vi "RP Lockin Fast Continuous Sweeper.vi"(6 "Samples per read":i32=1024, 7 "Desimate result":i32, 8 "Error In":errorcluster, 9 "milliseconds to wait":u32=10, 10 "Frequencies":dbl[](array[numeric]), 11 "connection ID":refnum<k5>) -> (0 "Error Out":errorcluster, 1 "Y":dbl[](array[numeric]), 2 "X":dbl[](array[numeric]), 3 "connection ID out":refnum<k5>, 4 "F":dbl[](array[numeric]))   [LabVIEW 2015]
panel:
  out "Input Fifo cnt 2":i32
  out "32bit integer":i32
  out "Output Fifo cnt":i32
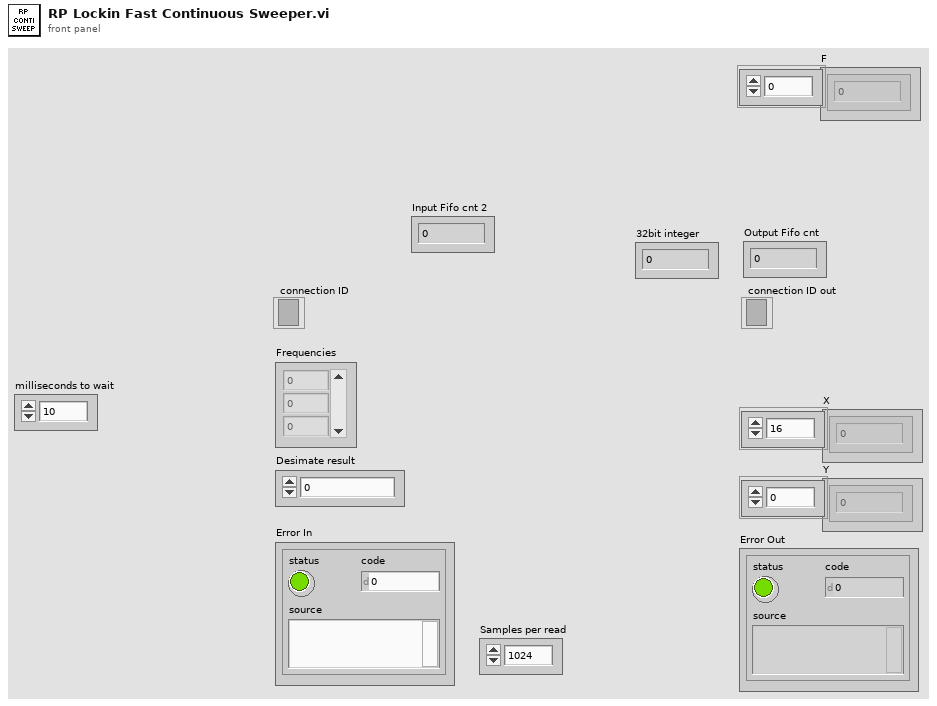
[diagram p1: front panel]
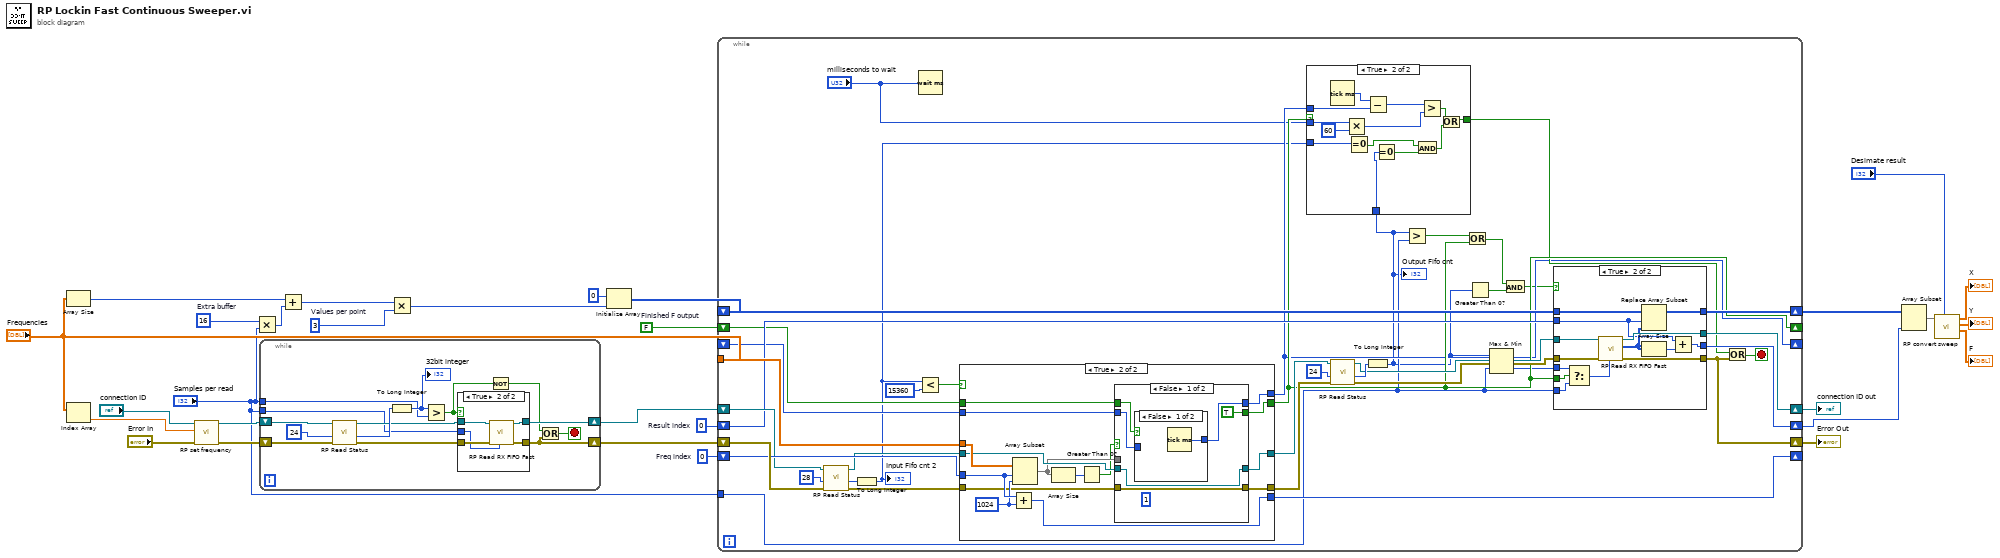
[diagram p0: block diagram]
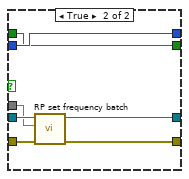
[diagram p6: hidden frame]
diagram:
  w13 = 3  # Values per point
  w16 = 16  # Extra buffer
  w19 = FALSE  # Finished F output
  w21 = 0  # Freq index
  w9 = 0  # Result index
  n1 = Array Size(array="Frequencies") -> (size(s)=w17:i32)
  n2 = Index Array(array="Frequencies") -> (element=w29:dbl)  [unwired: 1 in]
  n3 = call "RP set frequency.vi"("Error In"="Error In", "Frequency"=w29, "connection ID"="connection ID") -> ("Error Out"=w23:errorcluster, "connection ID out"=w25:refnum<k5>)  [unwired: 6 in, 1 out]
  n4 = Multiply(x=w16, y="Samples per read") -> (x*y=w15:i32)
  n5 = while {
    tunnel: "Samples per read" -> [w40]
    shift-right: [w30] -> w22
    shift-left: w23 -> [w37]
    shift-right: [w35] -> w24
    shift-left: w25 -> [w36]
    tunnel: "Samples per read" -> [w34]
    stop <- w33 stop-if-true
    n6 = call "RP Read Status.vi"("Error In"=w37, "Status offset"=u64 24, "connection ID"=w36) -> ("Error Out"=w32:errorcluster, "Status response"=w41:u32, "connection ID out"=w39:refnum<k5>)  [unwired: 6 in]
    n7 = To Long Integer(number=w41) -> (32bit integer=w42:i32)
    "32bit integer" <- w42
    n8 = Greater?(x=w42, y=w40) -> (0:w38:bool)
    n9 = case shown="True" w38 {
      tunnel: w39 -> [w45 w50]
      tunnel: w32 -> [w44 w49]
      tunnel: [w44 w48] -> w30
      tunnel: [w45 w47] -> w35
      tunnel: w34 -> [_ w46]
      frame False {
      }
      frame True {
        n10 = call "RP Read RX FIFO Fast.vi"("Samples per read"=w46, "Error In"=w49, "connection ID"=w50) -> ("Error Out"=w48:errorcluster, "connection ID out"=w47:refnum<k5>)  [unwired: 6 in, 1 out]
      }
    }
    n11 = Not(x=w38) -> (.not. x?=w31:bool)
    n12 = Or(x=w31, y=w30) -> (x .or. y?=w33:bool)
  }
  n13 = Add(x=w17, y=w15) -> (x+y=w14:i32)
  n14 = Multiply(x=w14, y=w13) -> (x*y=w11:i32)
  n15 = Initialize Array(0, w11) -> (w10:i32[])
  n16 = while {
    tunnel: "Frequencies" -> [w88]
    tunnel: "Samples per read" -> [w54]
    shift-right: [w63] -> w20
    shift-left: w22 -> [w87]
    shift-right: [w86] -> w26
    shift-left: w24 -> [w70]
    shift-right: [w83] -> _
    shift-left: w21 -> [w84]
    shift-right: [w60] -> _
    shift-left: w19 -> [w61]
    shift-right: [w66] -> w8
    shift-left: w10 -> [w69]
    shift-right: [w67] -> w5
    shift-left: w9 -> [w68]
    shift-right: [w58] -> _
    shift-left: _ -> [w62]
    stop <- w85 stop-if-true
    n17 = call "RP Read Status.vi"("Error In"=w87, "Status offset"=u64 28, "connection ID"=w70) -> ("Error Out"=w74:errorcluster, "Status response"=w78:u32, "connection ID out"=w73:refnum<k5>)  [unwired: 6 in]
    n18 = To Long Integer(number=w78) -> (32bit integer=w52:i32)
    "Input Fifo cnt 2" <- w52
    n19 = Wait (ms)(milliseconds to wait="milliseconds to wait") -> ()  [unwired: 1 out]
    n20 = Less?(x=w52, y=15360) -> (x < y?=w75:bool)
    n21 = case shown="True" w75 {
      tunnel: w84 -> [w107 w121]
      tunnel: w88 -> [_ w122]
      tunnel: [w107 w119] -> w83
      tunnel: w74 -> [w105 w117]
      tunnel: w73 -> [w106 w116]
      tunnel: [w106 w115] -> w72
      tunnel: [w105 w114] -> w71
      tunnel: [w104 w111] -> w58
      tunnel: w62 -> [w104 w110]
      tunnel: w61 -> [w103 w109]
      tunnel: [w103 w108] -> w60
      frame False {
      }
      frame True {
        w120 = 1024
        n22 = Add(x=w121, y=w120) -> (x+y=w119:i32)
        n23 = Array Subset(array=w122, index=w121, length=w120) -> (w113:dbl[])
        n24 = Array Size(array=w113) -> (size(s)=w118:i32)
        n25 = Greater Than 0?(x=w118) -> (x > 0?=w112:bool)
        n26 = case shown="False" w112 {
          tunnel: w117 -> [w128 w137]
          tunnel: w116 -> [w127 w136]
          tunnel: [w127 w135] -> w115
          tunnel: [w128 w134] -> w114
          tunnel: w113 -> [_ w133]
          tunnel: [w126 w132] -> w111
          tunnel: w110 -> [w125 w132]
          tunnel: w109 -> [w124 w131]
          tunnel: [TRUE w131] -> w108
          frame False {
            (unwired) 1
            n27 = case shown="False" w124 {
              tunnel: [w129 w130] -> w126
              tunnel: w125 -> [_ w130]
              frame False {
                n28 = Tick Count (ms)() -> (millisecond timer value=w129:u32)
              }
              frame True {
              }
            }
          }
          frame True {
            n29 = call "RP set frequency batch.vi"("Error In"=w137, "Frequency"=w133, "connection ID"=w136) -> ("Error Out"=w134:errorcluster, "connection ID out"=w135:refnum<k5>)  [unwired: 7 in]
          }
        }
      }
    }
    n30 = call "RP Read Status.vi"("Error In"=w71, "Status offset"=u64 24, "connection ID"=w72) -> ("Error Out"=w79:errorcluster, "Status response"=w81:u32, "connection ID out"=w80:refnum<k5>)  [unwired: 6 in]
    n31 = To Long Integer(number=w81) -> (32bit integer=w53:i32)
    "Output Fifo cnt" <- w53
    n32 = case shown="True" w60 {
      selector: w60 -> [w89 _]
      tunnel: [w89 w94] -> w59
      tunnel: w58 -> [_ w99]
      tunnel: w53 -> [_ w98]
      tunnel: w52 -> [_ w97]
      tunnel: "milliseconds to wait" -> [_ w92]
      frame False {
      }
      frame True {
        n33 = Tick Count (ms)() -> (millisecond timer value=w101:u32)
        n34 = Multiply(x=w92, y=u32 60) -> (x*y=w90:u32)
        n35 = Equal To 0?(x=w97) -> (x = 0?=w96:bool)
        n36 = Subtract(x=w101, y=w99) -> (x-y=w102:u32)
        n37 = Equal To 0?(x=w98) -> (x = 0?=w95:bool)
        n38 = And(x=w96, y=w95) -> (x .and. y?=w93:bool)
        n39 = Greater?(x=w102, y=w90) -> (0:w100:bool)
        n40 = Or(x=w100, y=w93) -> (x .or. y?=w94:bool)
      }
    }
    n41 = Greater?(x=w53, y=w54) -> (0:w64:bool)
    n42 = Or(x=w64, y=w60) -> (x .or. y?=w65:bool)
    n43 = Greater Than 0?(x=w53) -> (x > 0?=w56:bool)
    n44 = Max & Min(x=w53, y=w54) -> (min(x,y)=w55:i32)  [unwired: 1 out]
    n45 = And(x=w65, y=w56) -> (x .and. y?=w57:bool)
    n46 = case shown="True" w57 {
      tunnel: w80 -> [w140 w155]
      tunnel: w79 -> [w141 w153]
      tunnel: [w141 w152] -> w63
      tunnel: [w140 w154] -> w86
      tunnel: w69 -> [w139 w151]
      tunnel: w68 -> [w138 w145]
      tunnel: [w138 w143] -> w67
      tunnel: [w139 w149] -> w66
      tunnel: w54 -> [_ w146]
      tunnel: w55 -> [_ w147]
      tunnel: w60 -> [_ w142]
      frame False {
      }
      frame True {
        n47 = Select(t=w147, s=w142, f=w146) -> (s? t:f=w148:i32)
        n48 = call "RP Read RX FIFO Fast.vi"("Samples per read"=w148, "Error In"=w153, "connection ID"=w155) -> ("Error Out"=w152:errorcluster, "FIFO out"=w150:i32[], "connection ID out"=w154:refnum<k5>)  [unwired: 6 in]
        n49 = Replace Array Subset(array=w151, new element=w150, index=w145) -> (w149:i32[])
        n50 = Array Size(array=w150) -> (size(s)=w144:i32)
        n51 = Add(x=w145, y=w144) -> (x+y=w143:i32)
      }
    }
    n52 = Or(x=w59, y=w63) -> (x .or. y?=w85:bool)
  }
  "connection ID out" <- w26
  "Error Out" <- w20
  n53 = Array Subset(array=w8, length=w5) -> (w6:i32[])  [unwired: 1 in]
  n54 = call "RP convert sweep.vi"("Desimate result"="Desimate result", "FIFO"=w6) -> ("F out"=→"F":dbl[], "Y out"=→"Y":dbl[], "X out"=→"X":dbl[])  [unwired: 7 in]
